vi "NI VeriStand - Hide Progress Dialog.vi"(8 "error in (no error)":errorcluster) -> (0 "error out":errorcluster)   [LabVIEW 2020, in "Custom Device API.lvlib"]
uses:
  <vilib>/NI VeriStand/Custom Device API/Custom Device API.lvlib
  a8eab07a-0ae9-4064-90bc-5b481464ec93.vi
  <vilib>/NI VeriStand/Custom Device API/Custom Device Offline Path.vi
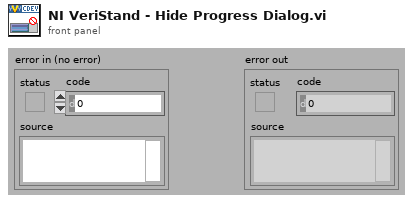
[diagram p1: front panel]
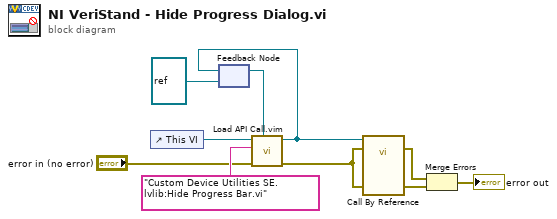
[diagram p0: block diagram]
diagram:
  n1 = control-ref of="This VI"() -> (w7:refnum<vi>)
  n2 = feedback #1(refnum<vi> refnum ("type specifier VI Refnum (for type only)")) -> (w8:refnum<vi>)
  n3 = call "Load API Call.vim"("VI reference in"=w8, "error in (no error)"="error in (no error)", "VI qualified name"="Custom Device Utilities SE.lvlib:Hide Progress Bar.vi", "Caller VI ref"=w7) -> ("error out"=w2:errorcluster, "VI reference"=w6:refnum<vi>)  [unwired: 6 in]
  n4 = feedback-in #1(w6) -> ()
  n5 = call-by-ref "?"(reference=w6, error in=w2, 8:"error in (no error)"=w2) -> (error out=w1:errorcluster, 0:"error out"=w10:errorcluster)  [unwired: 10 in, 1 out]
  n6 = Merge Errors(w1, w10) -> (→"error out":errorcluster)
